vi "Set speed.vi"(10 "speed":dbl, 11 "intake in":refnum<class "intake.lvclass">) -> (3 "intake out":refnum<class "intake.lvclass">)   [LabVIEW 2015]
uses:
  Robot Global Data.vi
  intake.lvclass
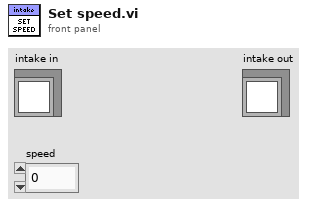
[diagram p1: front panel]
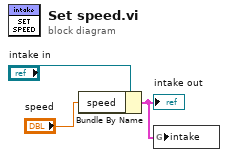
[diagram p0: block diagram]
diagram:
  n1 = Bundle By Name(cluster="intake in", "speed"="speed") -> (w1:cluster{})
  "intake out" <- w1
  n2 = global write "Robot Global Data.vi" "intake"(w1) -> ()
